vi "fromXml.vi"(8 "error in (no error)":errorcluster, 10 "dataPointXml":refnum<class "xmlNode.lvclass">, 11 "RampEvent in":refnum<class "RampEvent.lvclass">) -> (0 "error out":errorcluster, 3 "RampEvent out":refnum<class "RampEvent.lvclass">)   [LabVIEW 2011, in "Tools.lvlib" / "Scripting.lvlib" / "RampEvent.lvclass"]
uses:
  RampEvent.lvclass
  xmlNode/xmlNode.lvclass
  ScriptEvent.lvclass
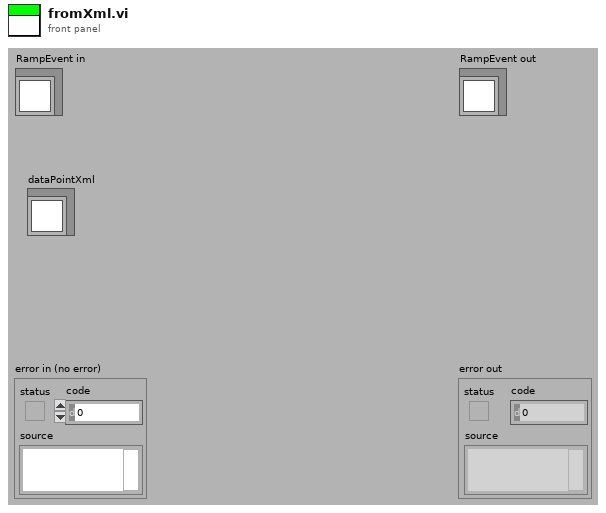
[diagram p1: front panel]
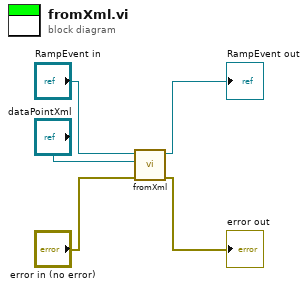
[diagram p0: block diagram]
diagram:
  n1 = call-parent "fromXml.vi"("error in (no error)"="error in (no error)", "dataPointXml"="dataPointXml", "ScriptEvent in"="RampEvent in") -> ("error out"=→"error out":errorcluster, "ScriptEvent out"=→"RampEvent out":refnum<class "RampEvent.lvclass">)  [unwired: 7 in]
